vi "Add Module to Project.vi"(7 "App Ref":refnum<vi>, 8 "error in":errorcluster, 11 "Library In":refnum<class "Library.lvclass">) -> (0 "error out":errorcluster, 3 "Library Out":refnum<class "Library.lvclass">)   [LabVIEW 2020, in "Panther Dashboard.lvlib" / "Library.lvclass"]
uses:
  Library.lvclass
  LabVIEWItem/Item Type--enum.ctl
  Library.lvclass/Library.ctl
  Read Library Ref.vi
  <vilib>/Delacor/Delacor QMH/Libraries/Scripting API/DQMH_Scripting API.lvlib
  LabVIEWItem/LabVIEWItem.lvclass
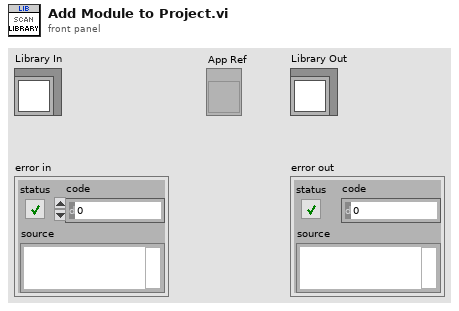
[diagram p1: front panel]
types:
  T1 = typedef "Panther Dashboard.lvlib/LabVIEWItem.lvclass/Item Type--enum.ctl" = enum16{"Requests", "Broadcasts", "Request and Wait for Reply", "Round Trip", "» Public API VIs", "» Constant VIs", "» Error VIs", "Module", "Project", "No Drag Selection"}
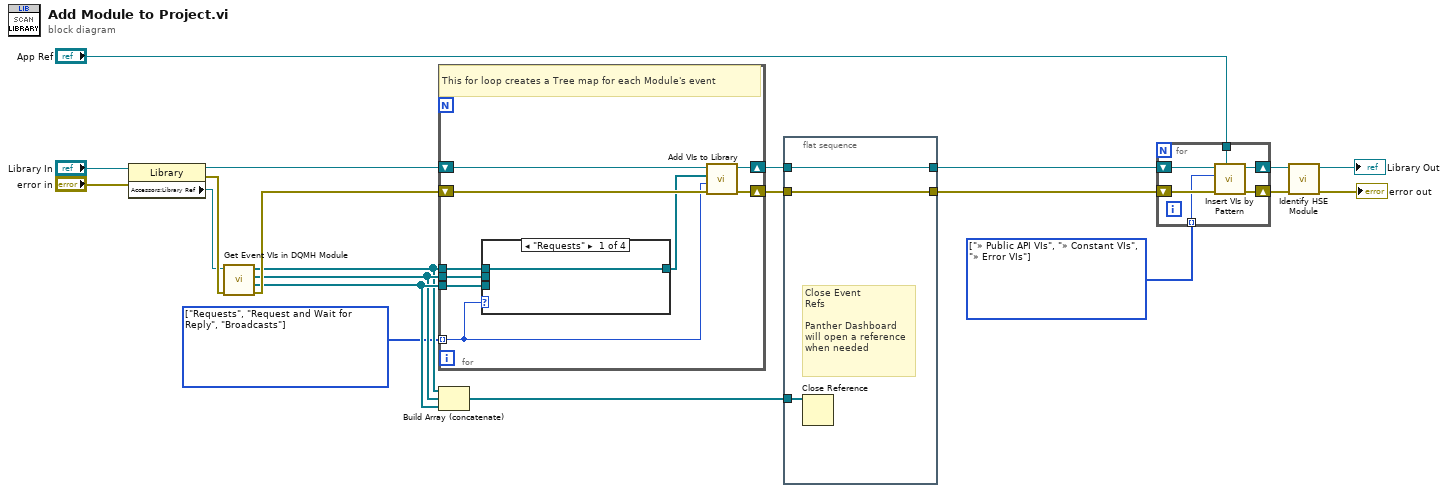
[diagram p0: block diagram]
diagram:
  w5 = T1[] [enum."» Public API VIs", enum."» Constant VIs", enum."» Error VIs"] items=["Requests", "Broadcasts", "Request and Wait for Reply", "Round Trip", "» Public API VIs", "» Constant VIs", "» Error VIs", "Module", "Project", "No Drag Selection"] ("Array")
  w6 = T1[] [enum."Requests", enum."Request and Wait for Reply", enum."Broadcasts"] items=["Requests", "Broadcasts", "Request and Wait for Reply", "Round Trip", "» Public API VIs", "» Constant VIs", "» Error VIs", "Module", "Project", "No Drag Selection"] ("Array")
  n1 = property class="Library"(reference="Library In", error in="error in") -> (reference out=w14:refnum<class "Library.lvclass">, error out=w21:errorcluster, "Accessors:Library Ref"=w13:refnum<vi>)
  n2 = call <vilib>:"Get Event VIs in DQMH Module.vi"("error in"=w21, "DQMH Module"=w13) -> ("error out"=w20:errorcluster, "Broadcast Event VIs"=w11:refnum<vi>[], "Request and Wait for Reply Event VIs"=w10:refnum<vi>[], "Request Event VIs"=w9:refnum<vi>[])  [unwired: 6 in]
  n3 = for {
    tunnel: w6 -> [w23] mode=indexing
    tunnel: w9 -> [w28]
    tunnel: w10 -> [w26]
    tunnel: w11 -> [w27]
    shift-right: [w24] -> w8
    shift-left: w14 -> [w25]
    shift-right: [w29] -> w18
    shift-left: w20 -> [w30]
    # "This for loop creates a Tree map for each Module's event"
    n4 = case shown="\"Requests\"" w23 {
      tunnel: w28 -> [w31 _ _ _]
      tunnel: w27 -> [_ _ _ w33]
      tunnel: w26 -> [_ _ w32 _]
      tunnel: [w31 _ w32 w33] -> w22
      frame "Requests" {
      }
      frame Default {
      }
      frame "Request and Wait for Reply" {
      }
      frame "Broadcasts" {
      }
    }
    n5 = call "Add VIs to Library.vi"("error in"=w30, "Event Type"=w23, "Event VIs"=w22, "Library In"=w25) -> ("error out"=w29:errorcluster, "Library Out"=w24:refnum<class "Library.lvclass">)  [unwired: 6 in]
  }
  n6 = Build Array (concatenate)(w9, w10, w11) -> (w12:refnum<vi>[])
  n7 = flat-sequence {
    tunnel: w12 -> [w35]
    tunnel: w8 -> [w34]
    tunnel: [w34] -> w7
    tunnel: w18 -> [w36]
    tunnel: [w36] -> w17
    frame #0 {
      # "Close Event\nRefs\n\nPanther Dashboard\nwill open a reference\nwhen needed"
      n8 = Close Reference(reference=w35) -> ()  [unwired: 1 in, 1 out]
    }
  }
  n9 = for {
    tunnel: "App Ref" -> [w40]
    shift-right: [w39] -> w4
    shift-left: w7 -> [w38]
    shift-right: [w41] -> w2
    shift-left: w17 -> [w42]
    tunnel: w5 -> [w37] mode=indexing
    n10 = call "Insert VIs by Pattern.vi"("Application in"=w40, "error in"=w42, "VI Type"=w37, "Library In"=w38) -> ("error out"=w41:errorcluster, "Library Out"=w39:refnum<class "Library.lvclass">)  [unwired: 6 in]
  }
  n11 = call "Identify HSE Module.vi"("error in"=w2, "Library in"=w4) -> ("error out"=→"error out":errorcluster, "Library out"=→"Library Out":refnum<class "Library.lvclass">)  [unwired: 8 in]
